vi "Initialize uWave Sensor.vi"(8 "error in (no error)":errorcluster, 9 "COM Port":refnum<visa-resource-name>, 10 "H3611i":bool, 11 "MWWL Verification in":refnum<class "MWWL Verification.lvclass">) -> (0 "error out":errorcluster, 3 "MWWL Verification out":refnum<class "MWWL Verification.lvclass">)   [LabVIEW 2018, in "MWWL Verification.lvlib" / "MWWL Verification.lvclass"]
uses:
  MWWL Verification.lvclass
  C:/Program Files (x86)/National Instruments/LabVIEW 2018/vi.lib/ActorFramework/Actor/Actor.lvclass
  MWWL Verification.lvclass/MWWL Verification.ctl
  H3611i Actor/H3611i Actor/H3611i Actor.lvclass
  Sensor Actor/Sensor Messages/Set Sensor COM Port Msg/Set Sensor COM Port Msg.lvclass/Set Sensor COM Port Msg.ctl
  <vilib>/ActorFramework/Message Enqueuer/Message Enqueuer.lvclass/Message Enqueuer.ctl
  H3611i Actor/H3611i Actor Messages/Configure H3611i Msg/Configure H3611i Msg.lvclass/Configure H3611i Msg.ctl
  <vilib>/ActorFramework/Message Enqueuer/Enqueue.vi
  Sensor Actor/Sensor Messages/Set Sensor COM Port Msg/Set Sensor COM Port Msg.lvclass
  C:/Program Files (x86)/National Instruments/LabVIEW 2018/vi.lib/ActorFramework/Message/Message.lvclass
  H3611i Actor/H3611i Actor Messages/Configure H3611i Msg/Configure H3611i Msg.lvclass
  <vilib>/ActorFramework/Message Priority Queue/Priority Enqueue.vi
  <vilib>/ActorFramework/Actor/Actor.lvclass
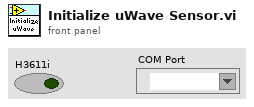
[diagram p1: front panel]
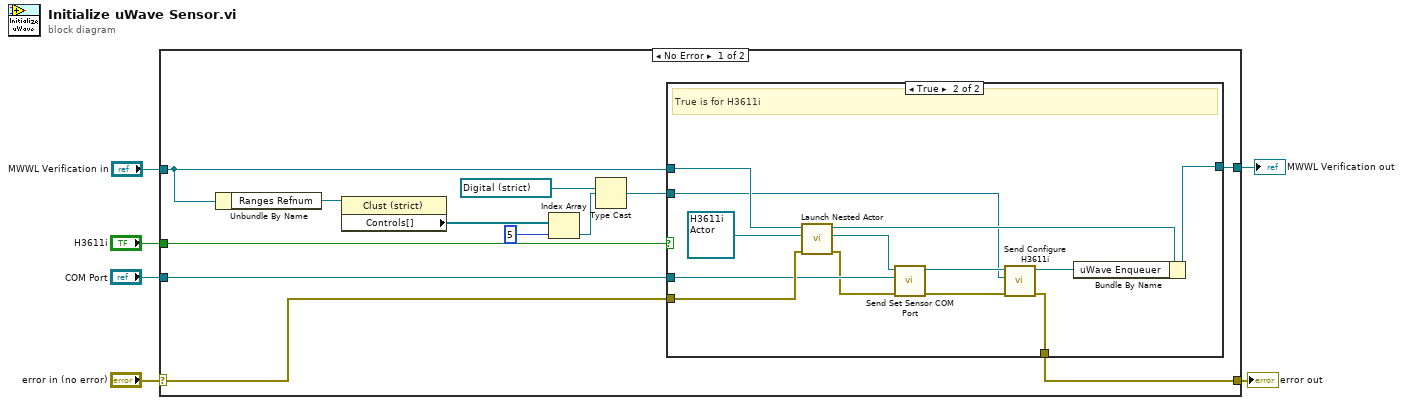
[diagram p0: block diagram]
diagram:
  n1 = case shown="No Error" "error in (no error)" {
    selector: "error in (no error)" -> [w16 w35]
    tunnel: [w15 w35] -> w5
    tunnel: [w17 w34] -> w2
    tunnel: "MWWL Verification in" -> [w13 w34]
    tunnel: "H3611i" -> [w18 _]
    tunnel: "COM Port" -> [w14 _]
    frame No Error {
      n2 = Unbundle By Name(w13) -> ("Ranges Refnum"=w9:refnum<vi>)
      n3 = property class="Clust (strict)"(reference=w9) -> ("Controls[]"=w10:refnum<vi>[])  [unwired: 1 in, 2 out]
      n4 = Index Array(array=w10, index=5) -> (element=w11:refnum<vi>)
      n5 = Type Cast(type=refnum<vi> refnum ("DLS Range Refnum"), x=w11) -> (*(type *) &x=w7:refnum<vi>)
      n6 = case shown="True" w18 {
        tunnel: w13 -> [w20 w22]
        tunnel: [w20 w32] -> w17
        tunnel: w16 -> [w19 w31]
        tunnel: [w19 w24] -> w15
        tunnel: w14 -> [_ w30]
        tunnel: w7 -> [_ w21]
        frame False {
          # "False is for Miros"
        }
        frame True {
          # "True is for H3611i"
          n7 = call <vilib>:"Launch Nested Actor.vi"("error in (no error)"=w31, "Nested Actor"=refnum<class "H3611i Actor.lvclass"> refnum ("H3611i.lvlib:H3611i Actor"), "Caller Actor in"=w22) -> ("error out"=w29:errorcluster, "Nested Actor's Enqueuer"=w28:refnum<class "Message Enqueuer.lvclass">, "Caller Actor out"=w23:refnum<class "MWWL Verification.lvclass">)  [unwired: 6 in]
          n8 = call "Send Set Sensor COM Port.vi"("error in (no error)"=w29, "COM Port"=w30, "Message Enqueuer in"=w28) -> ("error out"=w25:errorcluster, "Message Enqueuer out"=w27:refnum<class "Message Enqueuer.lvclass">)  [unwired: 7 in]
          n9 = call "Send Configure H3611i.vi"("error in (no error)"=w25, "uWave Range Refnum"=w21, "Message Enqueuer in"=w27) -> ("error out"=w24:errorcluster, "Message Enqueuer out"=w26:refnum<class "Message Enqueuer.lvclass">)  [unwired: 7 in]
          n10 = Bundle By Name(cluster=w23, "uWave Enqueuer"=w26) -> (w32:refnum<class "MWWL Verification.lvclass">)
        }
      }
    }
    frame Error {
    }
  }
  "error out" <- w5
  "MWWL Verification out" <- w2
